vi "MDPtr SetCopyCount.vi"(8 "Copy Count":i32, 9 "error in (no error)":errorcluster, 10 "HexStrPtr":T1) -> (2 "error out":errorcluster, 3 "HexStrPtr (dup)":T1)   [LabVIEW 2017, in "MDPtr.lvlib"]
uses:
  MDPtr.lvlib
  MDPtr TypeDef/MDPtr.ctl
  _Support/Error Handler/_Build Error Cluster.vi
  _MDPtrMgr/MDPtrMgr.lvclass
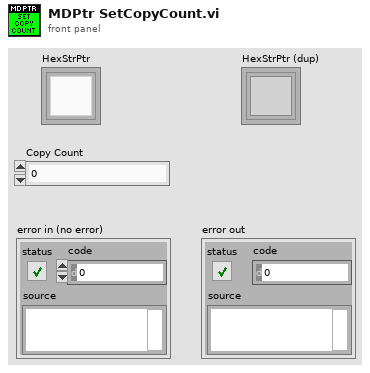
[diagram p1: front panel]
types:
  T1 = typedef "MDPtr.lvlib/MDPtr.ctl" = refnum<k1>
  T2 = typedef "MDPtr.lvlib/MDPtr DataFrame-Memory.ctl" = cluster{"Common":T3, "DVR":refnum<data-value>}
  T3 = typedef "MDPtr.lvlib/MDPtr DataFrame-Common.ctl" = cluster{"Data Type":T4, "Copy Count":i32, "String Attribute":string, "Cache Length":i32, "Data Length":i32}
  T4 = typedef "NI_Data Type.lvlib/Data Type.ctl" = enum8{"Invalid Type", "Void", "I8", "I16", "I32", "I64", "U8", "U16", "U32", "U64", "Single Float", "Double Float", "Extended Float", "Single Complex", "Double Complex", "Extended Complex", "Enum U8", "Enum U16", "Enum U32", "Enum U64", "Single Float With Unit", "Double Float With Unit", "Extended Float With Unit", "Single Complex with Unit", "Double Complex with Unit", "Extended Complex with Unit", "Boolean", "String", "Path", "Picture", "Tag", "Array", "Cluster", "Variant", "LV Variant", "Waveform", "Timestamp", "Digital Waveform", "Digital Data", "ExpressData", "Refnum", "External Data", "VI", "Poly VI", "LabVIEW Class Instance", "Fixed Point"}
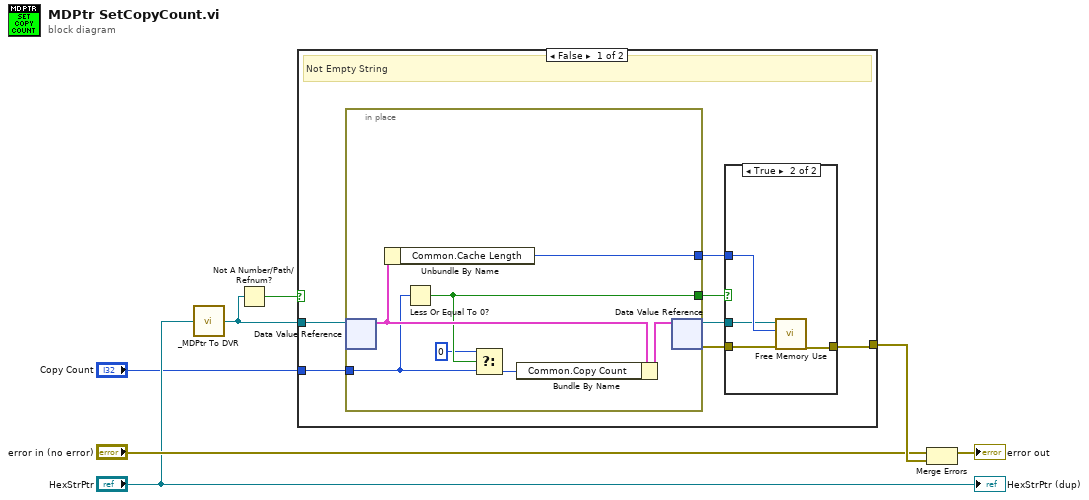
[diagram p0: block diagram]
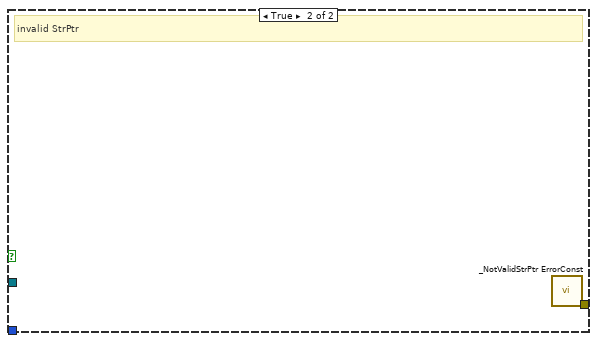
[diagram p3: hidden frame]
diagram:
  n1 = call "_MDPtr To DVR.vi"("MDPtr"="HexStrPtr") -> ("MDPtr DVR"=w2:refnum<data-value>)
  n2 = Not A Number/Path/Refnum?(number/path/refnum=w2) -> (NaN/Path/Refnum?=w3:bool)
  n3 = case shown="False" w3 {
    tunnel: [w9 w27] -> w7
    tunnel: w2 -> [w14 _]
    tunnel: "Copy Count" -> [w13 _]
    frame False {
      # "Not Empty String"
      n4 = in-place {
        in-place-border: w13 -> [w21]
        in-place-border: [w23] -> w11
        in-place-border: [w24] -> w8
        n5 = in-place-dvr #1(w14) -> (w25:T2)  [unwired: 1 out]
        n6 = Unbundle By Name(w25) -> ("Common.Cache Length"=w24:i32)
        n7 = Less Or Equal To 0?(x=w21) -> (x <= 0?=w23:bool)
        n8 = Select(t=0, s=w23, f=w21) -> (s? t:f=w20:i32)
        n9 = Bundle By Name(cluster=w25, "Common.Copy Count"=w20) -> (w26:T2)
        n10 = in-place-dvr #1(w26) -> (w12:refnum<data-value>, w10:errorcluster)
      }
      n11 = case shown="True" w11 {
        tunnel: [w15 w19] -> w9
        tunnel: w8 -> [_ w18]
        tunnel: w10 -> [w15 w17]
        tunnel: w12 -> [_ w16]
        frame False {
        }
        frame True {
          n12 = call "Free Memory Use.vi"("error in"=w17, "Cache Length"=w18, "MDPtr DVR"=w16) -> ("error out"=w19:errorcluster)  [unwired: 8 in]
        }
      }
    }
    frame True {
      # "invalid StrPtr"
      n13 = call "_NotValidStrPtr ErrorConst.vi"() -> ("error out"=w27:errorcluster)  [unwired: 19 in]
    }
  }
  n14 = Merge Errors("error in (no error)", w7) -> (→"error out":errorcluster)
  "HexStrPtr (dup)" <- "HexStrPtr"
